vi "Get image with missed frame check.vi"(8 "error in":errorcluster, 11 "Control IN":T1={"Core"={"Current VI Reference"=refnum, "Close Panel on Exit?"=FALSE}, "IA JSON File Path"=path "", "Buffer Number"=0, "Missed Frame Count"=-1, "Timeout"=0, "Image_Counter_CA"=0, "Imaqdx Session In"="", "filenames"=[], "File path to read images"=path "", "Sequence"="", "IMAQ ring Buffer"=[], "Buffer count"=0, "AOI"=[], "Offline Images Ring Buffer"=[], "ReceiverSequence"=[], "Number Of Buffers"=0, "IMAQ Offline Image Buffer"=[], "IMAQ Run image Buffer "=[], "Camera parameters"={"Camera parameters"={"Id"=0, "Type"="", "Model"="", "InterfaceType"="", "SerialNumber"="", "Timeout"=0, "NumberOfBuffers"=0, "AcquisitionTimeout"=0, "ImageName"="", "ColorCameraParam"={"PixelFormat"="", "GammaEnable"=FALSE, "GammaSelector"="", "BalanceRationSelector"=[], "BalanceRationRaw"=[], "BalanceWhiteAuto"="", "LightSourceSelector"=""}, "sessionID"="", "Continuous?"=enum."One Shot", "Image Type"=0, "Buffer Number Mode (Next)"=enum."Next", "PartsList"=[{"Name"="", "ReceiverSequence"=[], "AOI"=[], "filePath"=""}], "AOI "=[], "Default file path"=path "", "Offline"=FALSE, "GeneralCameraConfig"=[], "DefaultReceiverSequence"=[], "Front Panel Open?"=FALSE}, "PartName"=[]}, "CurrentPartParameters"={"Name"="", "ReceiverSequence"=[], "AOI"=[], "filePath"=""}, "Exposure Time"=0, "File path @ Run"=path "", "State Ack"={"State"="", "Status"=""}} {"Camera parameters"."Camera parameters"."Image Type" items=["Grayscale (U8)", "Grayscale (I16)", "Grayscale (SGL)", "Complex (CSG)", "RGB (U32)", "HSL (U32)", "RGB (U64)", "Grayscale (U16)"]}) -> (0 "error out":errorcluster, 2 "Get image Cluster":T8, 3 "Controls Out":T1={"Core"={"Current VI Reference"=refnum, "Close Panel on Exit?"=FALSE}, "IA JSON File Path"=path "", "Buffer Number"=0, "Missed Frame Count"=-1, "Timeout"=0, "Image_Counter_CA"=0, "Imaqdx Session In"="", "filenames"=[], "File path to read images"=path "", "Sequence"="", "IMAQ ring Buffer"=[], "Buffer count"=0, "AOI"=[], "Offline Images Ring Buffer"=[], "ReceiverSequence"=[], "Number Of Buffers"=0, "IMAQ Offline Image Buffer"=[], "IMAQ Run image Buffer "=[], "Camera parameters"={"Camera parameters"={"Id"=0, "Type"="", "Model"="", "InterfaceType"="", "SerialNumber"="", "Timeout"=0, "NumberOfBuffers"=0, "AcquisitionTimeout"=0, "ImageName"="", "ColorCameraParam"={"PixelFormat"="", "GammaEnable"=FALSE, "GammaSelector"="", "BalanceRationSelector"=[], "BalanceRationRaw"=[], "BalanceWhiteAuto"="", "LightSourceSelector"=""}, "sessionID"="", "Continuous?"=enum."One Shot", "Image Type"=0, "Buffer Number Mode (Next)"=enum."Next", "PartsList"=[{"Name"="", "ReceiverSequence"=[], "AOI"=[], "filePath"=""}], "AOI "=[], "Default file path"=path "", "Offline"=FALSE, "GeneralCameraConfig"=[], "DefaultReceiverSequence"=[], "Front Panel Open?"=FALSE}, "PartName"=[]}, "CurrentPartParameters"={"Name"="", "ReceiverSequence"=[], "AOI"=[], "filePath"=""}, "Exposure Time"=0, "File path @ Run"=path "", "State Ack"={"State"="", "Status"=""}} {"Camera parameters"."Camera parameters"."Image Type" items=["Grayscale (U8)", "Grayscale (I16)", "Grayscale (SGL)", "Complex (CSG)", "RGB (U32)", "HSL (U32)", "RGB (U64)", "Grayscale (U16)"]})   [LabVIEW 2019, in "Image Acquisition.lvlib" / "Image Acquisition.lvclass"]
doc: "camera image acquision"
uses:
  Image Acquisition.lvclass
  <vilib>/vision/Image Controls.llb/IMAQ Image.ctl
  TypeDefs/Acquired Image Info.ctl
  <vilib>/userdefined/High Color/IMAQdx.ctl
  <vilib>/vision/driver/IMAQdx.llb/IMAQdx Buffer Number Mode.ctl
  <vilib>/vision/driver/IMAQdx.llb/IMAQdx Acquisition Mode.ctl
  TypeDefs/Image Acquisition Parameters.ctl
  TypeDefs/Initialize Data IA.ctl
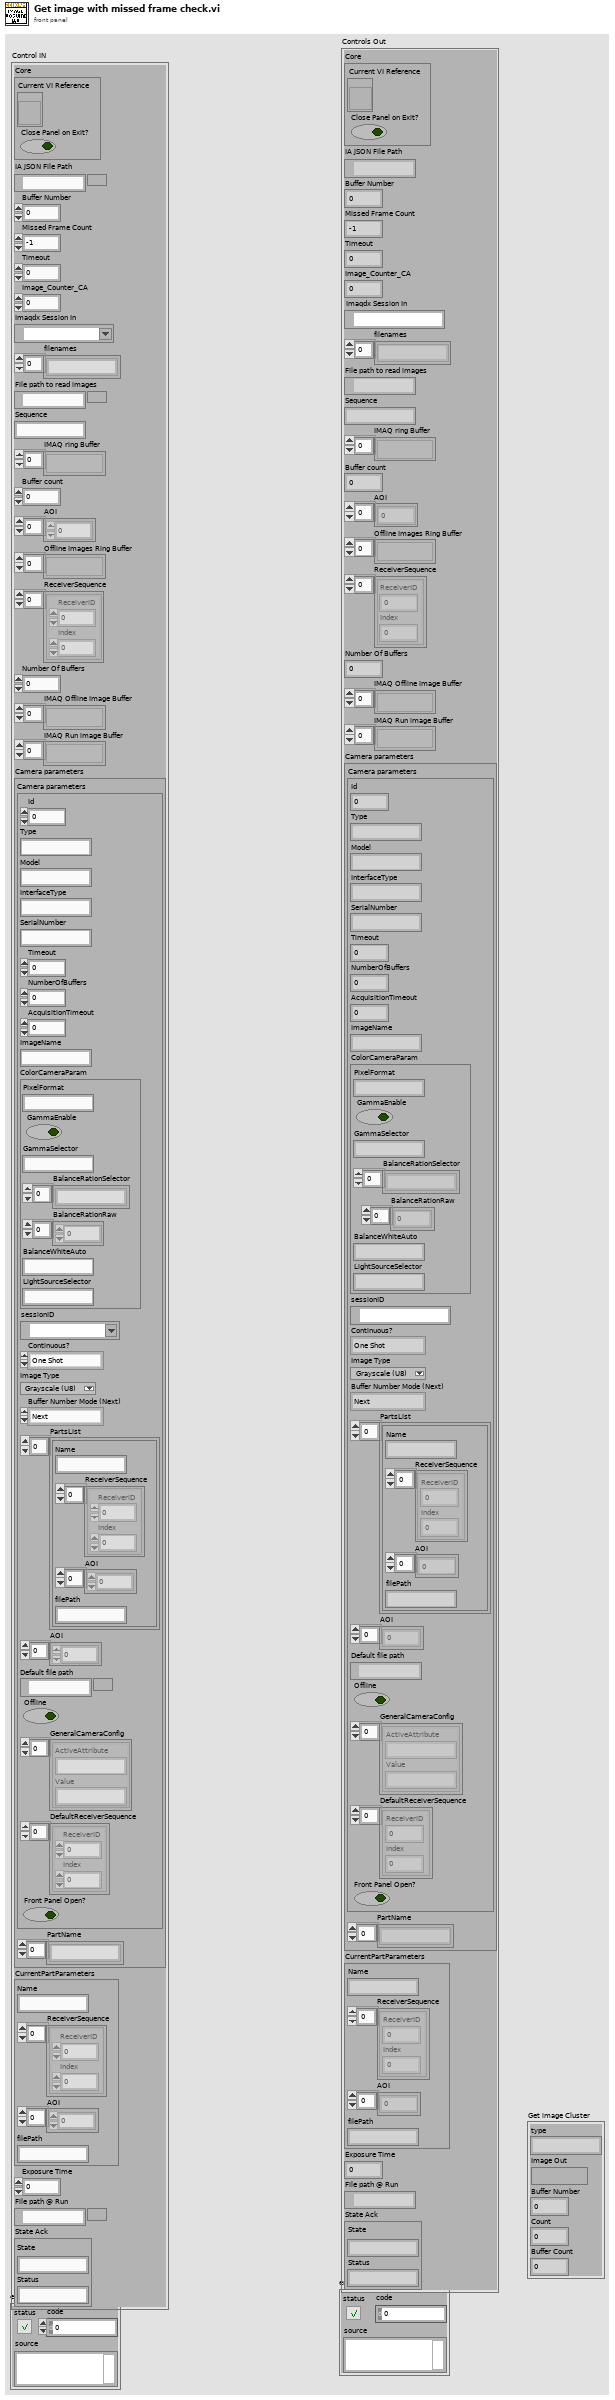
[diagram p1: front panel]
types:
  T1 = typedef "Image Acquisition.lvlib/Image Acquisition.lvclass/Initialize Data IA.ctl" = cluster{"Core":cluster{"Current VI Reference":refnum<vi>, "Close Panel on Exit?":bool}, "IA JSON File Path":path, "Buffer Number":u64, "Missed Frame Count":i32, "Timeout":i32, "Image_Counter_CA":u64, "Imaqdx Session In":T2, "filenames":string[], "File path to read images":path, "Sequence":string, "IMAQ ring Buffer":T3[], "Buffer count":i32, "AOI":i32[], "Offline Images Ring Buffer":T3[], "ReceiverSequence":cluster{"ReceiverID":i32, "Index":i32}[], "Number Of Buffers":i32, "IMAQ Offline Image Buffer":T3[], "IMAQ Run image Buffer ":T3[], "Camera parameters":T4, "CurrentPartParameters":cluster{"Name":string, "ReceiverSequence":cluster{"ReceiverID":dbl, "Index":dbl}[], "AOI":i32[], "filePath":string}, "Exposure Time":u32, "File path @ Run":path, "State Ack":cluster{"State":string, "Status":string}}
  T2 = typedef "IMAQdx.ctl" = refnum<k21>
  T3 = typedef "IMAQ Image.ctl" = refnum<image>
  T4 = typedef "Image Acquisition.lvlib/Image Acquisition.lvclass/Image Acquisition Parameters.ctl" = cluster{"Camera parameters":cluster{"Id":i32, "Type":string, "Model":string, "InterfaceType":string, "SerialNumber":string, "Timeout":i32, "NumberOfBuffers":i32, "AcquisitionTimeout":i32, "ImageName":string, "ColorCameraParam":cluster{"PixelFormat":string, "GammaEnable":bool, "GammaSelector":string, "BalanceRationSelector":string[], "BalanceRationRaw":i32[], "BalanceWhiteAuto":string, "LightSourceSelector":string}, "sessionID":T2, "Continuous?":T5, "Image Type":T6, "Buffer Number Mode (Next)":T7, "PartsList":cluster{"Name":string, "ReceiverSequence":cluster{"ReceiverID":dbl, "Index":dbl}[], "AOI":i32[], "filePath":string}[], "AOI ":i32[], "Default file path":path, "Offline":bool, "GeneralCameraConfig":cluster{"ActiveAttribute":string, "Value":string}[], "DefaultReceiverSequence":cluster{"ReceiverID":dbl, "Index":dbl}[], "Front Panel Open?":bool}, "PartName":string[]}
  T5 = typedef "NI_Vision_Acquisition_Software.lvlib/IMAQdx Acquisition Mode.ctl" = enum32{"One Shot", "Continuous"}
  T6 = typedef "Image Type" = u32
  T7 = typedef "NI_Vision_Acquisition_Software.lvlib/IMAQdx Buffer Number Mode.ctl" = enum32{"Next", "Last", "Buffer Number", "Every", "Last New"}
  T8 = typedef "Image Acquisition.lvlib/Image Acquisition.lvclass/Acquired Image Info.ctl" = cluster{"type":string, "Image Out":T3, "Buffer Number":u64, "Count":u64, "Buffer Count":u64}
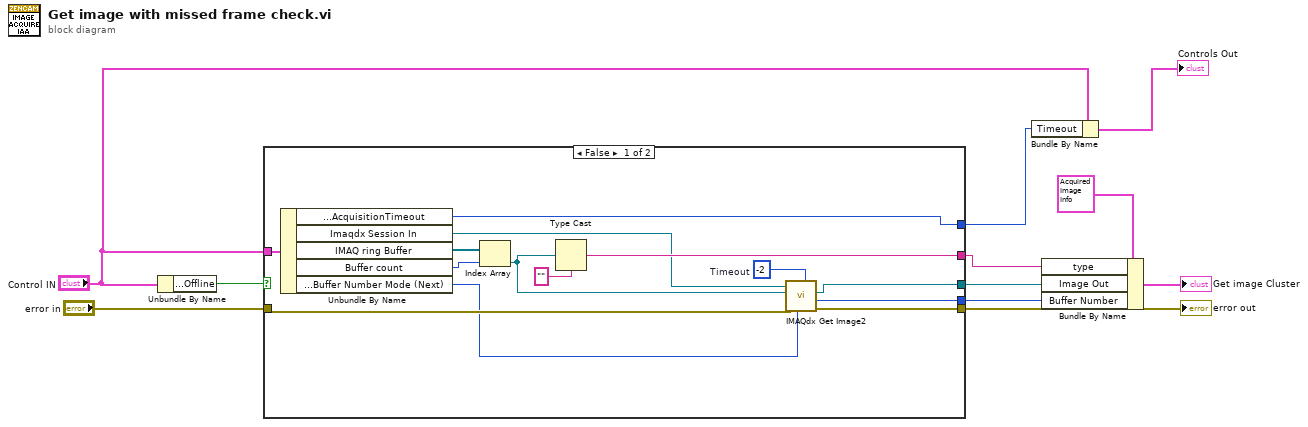
[diagram p0: block diagram]
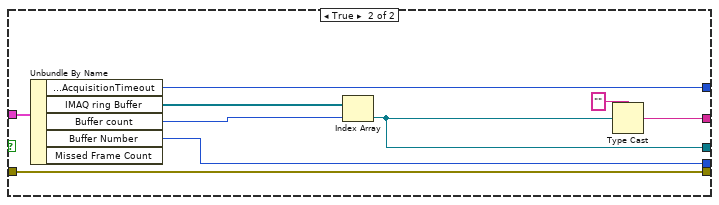
[diagram p2: hidden frame]
diagram:
  n1 = Unbundle By Name("Control IN") -> ("Camera parameters.Camera parameters.Offline"=w10:bool)
  n2 = case shown="False" w10 {
    tunnel: "Control IN" -> [w23 w33]
    tunnel: "error in" -> [w21 w31]
    tunnel: [w25 w31] -> w9
    tunnel: [w24 w28] -> w7
    tunnel: [w19 w29] -> w8
    tunnel: [w14 w32] -> w6
    tunnel: [w12 w26] -> w1
    frame False {
      w15 = -2  # Timeout
      n3 = Unbundle By Name(w23) -> ("Camera parameters.Camera parameters.AcquisitionTimeout"=w12:i32, "Imaqdx Session In"=w16:T2, "IMAQ ring Buffer"=w22:T3[], "Buffer count"=w17:i32, "Camera parameters.Camera parameters.Buffer Number Mode (Next)"=w13:T7)
      n4 = Index Array(array=w22, index=w17) -> (element=w20:T3)
      n5 = Type Cast(type="", x=w20) -> (*(type *) &x=w19:string)
      n6 = call <vilib>:"IMAQdx Get Image2.vi"("Timeout (ms)"=w15, "Buffer Number Mode (Next)"=w13, "error in"=w21, "Image In"=w20, "Session In"=w16) -> ("error out"=w25:errorcluster, "Buffer Number Out"=w14:u32, "Image Out"=w24:T3)  [unwired: 3 in, 1 out]
    }
    frame True {
      n7 = Unbundle By Name(w33) -> ("Camera parameters.Camera parameters.AcquisitionTimeout"=w26:i32, "IMAQ ring Buffer"=w34:T3[], "Buffer count"=w27:i32, "Buffer Number"=w32:u64)  [unwired: 1 out]
      n8 = Index Array(array=w34, index=w27) -> (element=w28:T3)
      n9 = Type Cast(type="", x=w28) -> (*(type *) &x=w29:string)
    }
  }
  "error out" <- w9
  n10 = Bundle By Name(cluster="Control IN", "Timeout"=w1) -> (→"Controls Out":T1)
  n11 = Bundle By Name(cluster=T8 {"type"="", "Image Out"=refnum, "Buffer Number"=0, "Count"=0, "Buffer Count"=0} ("Get image cluster out"), "type"=w8, "Image Out"=w7, "Buffer Number"=w6) -> (→"Get image Cluster":T8)
